vi "Colour JSON items in a string control.vi"() -> ()   [LabVIEW 2019]
doc: "Shows how to colour the individual JSON elements using JSONtext."
uses:
  vi.lib/JDP Science/JSONtext/JSONtext.lvlib
panel:
  out "error out":errorcluster
  out "JSON (coloured)":string
  in  "JSON":string="{\r        \"sequence\":22222222,\r        \"prev_out\":{\r          \"spent\":true,\r          \"tx_index\":99005469,\r          \"type\":1,\r          \"addr\":\"Blah Blah Blah\",\r          \"value\":1,\r          \"n\":0,\r          \"script\":\"76a91477f4c9ee75e449a74c21a\",\n          \"array\":[12,34,56,[1,2,3],78,\"a\",\"b\",\"c\",123,true,true,false]\r}"
  # "Run this VI"
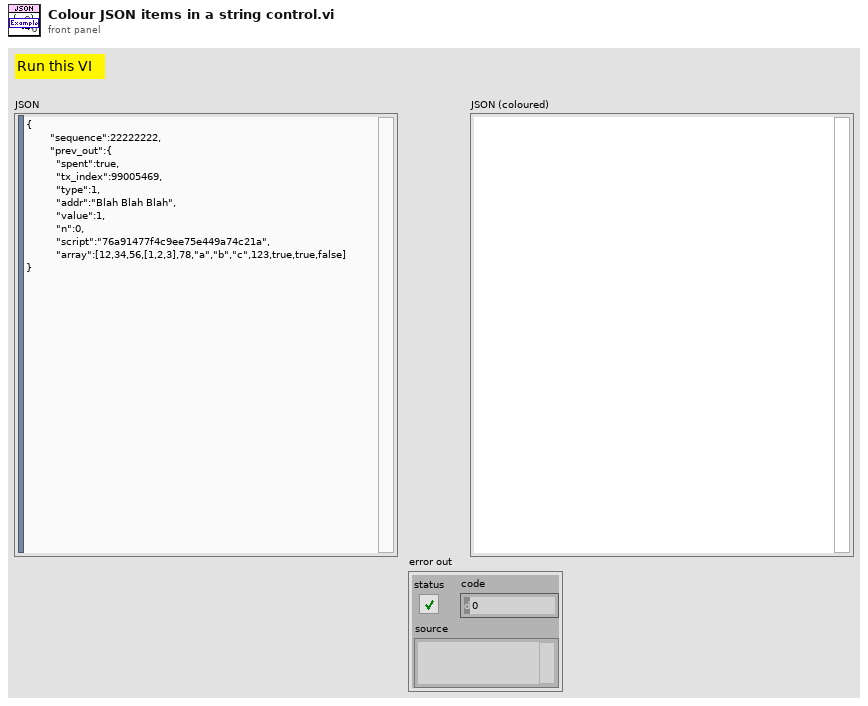
[diagram p1: front panel]
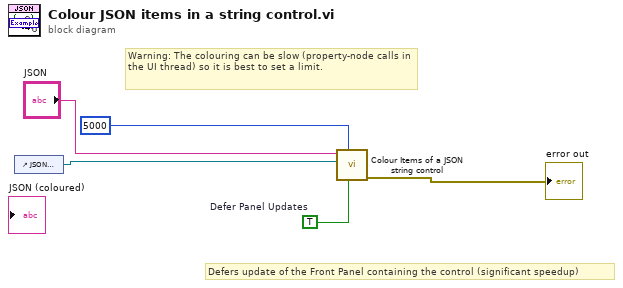
[diagram p0: block diagram]
diagram:
  w1 = TRUE  # Defer Panel Updates
  # "Defers update of the Front Panel containing the control (significant speedup)"
  # "Warning: The colouring can be slow (property-node calls in the UI thread) so it is best to set a limit."
  n1 = control-ref of="JSON (coloured)"() -> (w2:refnum<vi>)
  n2 = call "Colour Items of a JSON string control.vi"("Defer Panel Updates"=w1, "Maximum UI Property calls"=5000, "String Control"=w2, "JSON"="JSON") -> ("error out"=→"error out":errorcluster)  [unwired: 7 in]
